vi "Write TDMS.vi"(8 "error in (no error)":errorcluster, 9 "Velocity (rad/Sec)":dbl, 10 "Angular Position (rad)":dbl, 11 "Maxon Encoder in":refnum<class "Maxon Encoder.lvclass">) -> (0 "error out":errorcluster, 3 "Maxon Encoder out":refnum<class "Maxon Encoder.lvclass">)   [LabVIEW 2019, in "Maxon Encoder.lvclass"]
doc: "Writes data to the tdms file. Call Open TDMS VI before running this VI."
uses:
  Maxon Encoder.lvclass
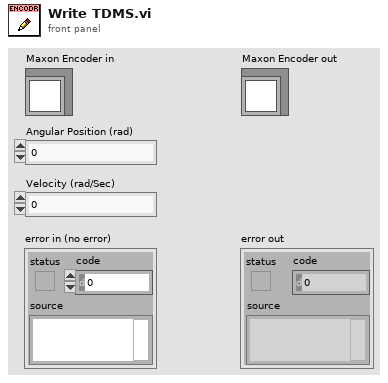
[diagram p1: front panel]
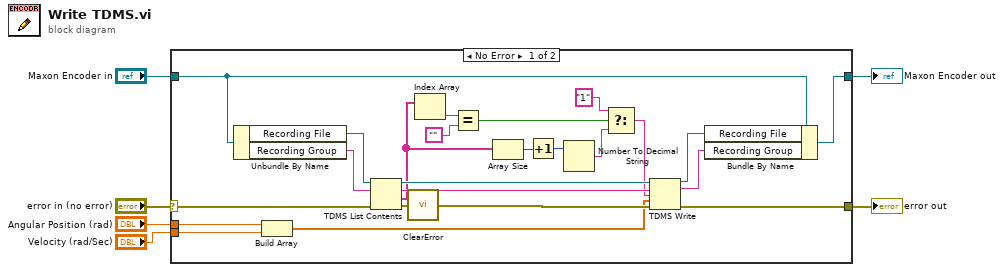
[diagram p0: block diagram]
diagram:
  n1 = case shown="No Error" "error in (no error)" {
    selector: "error in (no error)" -> [w23 w32]
    tunnel: [w30 w32] -> w2
    tunnel: [w26 w31] -> w1
    tunnel: "Maxon Encoder in" -> [w29 w31]
    tunnel: "Angular Position (rad)" -> [w9 _]
    tunnel: "Velocity (rad/Sec)" -> [w8 _]
    frame No Error {
      n2 = Unbundle By Name(w29) -> ("Recording File"=w25:refnum<k34>, "Recording Group"=w24:string)
      n3 = Build Array(w9, w8) -> (w10:dbl[])
      n4 = TDMS List Contents(4:w23, 6:w24, 7:w25) -> (0:w7:errorcluster, 1:w13:string[], 2:w22:string, 3:w21:refnum<k34>)
      n5 = call <vilib>:"ClearError.vi"("error in (no error)"=w7) -> ("error out"=w18:errorcluster)
      n6 = Index Array(array=w13) -> (element=w17:string)  [unwired: 1 in]
      n7 = Equal?(x=w17, y="") -> (x = y?=w15:bool)
      n8 = Array Size(array=w13) -> (size(s)=w20:i32)
      n9 = Increment(x=w20) -> (x+1=w19:i32)
      n10 = Number To Decimal String(number=w19) -> (decimal integer string=w12:string)  [unwired: 1 in]
      n11 = Select(t="1", s=w15, f=w12) -> (s? t:f=w11:string)
      n12 = TDMS Write(0:w21, 5:w22, 7:w11, 9:w10, 11:w18) -> (4:w28:refnum<k34>, 6:w27:string, 15:w30:errorcluster)  [unwired: 1 in, 1 out]
      n13 = Bundle By Name(cluster=w29, "Recording File"=w28, "Recording Group"=w27) -> (w26:refnum<class "Maxon Encoder.lvclass">)
    }
    frame Error {
    }
  }
  "error out" <- w2
  "Maxon Encoder out" <- w1
